vi "send_tmr2_rld.vi"(2 "error in (no error)":errorcluster, 3 "frekvencia":u16, 4 "VISA Refnum in":refnum<visa-resource-name>) -> (0 "error out":errorcluster, 1 "VISA Refnum out":refnum<visa-resource-name>)   [LabVIEW 2013]
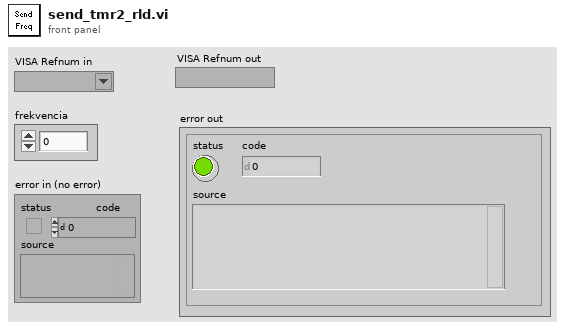
[diagram p1: front panel]
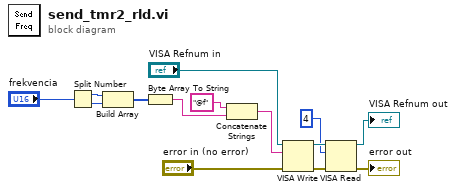
[diagram p0: block diagram]
diagram:
  n1 = Split Number(x="frekvencia") -> (hi(x)=w11:u8, lo(x)=w12:u8)
  n2 = Build Array(w11, w12) -> (w13:u8[])
  n3 = Byte Array To String(unsigned byte array=w13) -> (string=w14:string)
  n4 = Concatenate Strings("@f" ("write buffer"), w14) -> (w4:string)
  n5 = VISA Write(VISA resource name="VISA Refnum in", write buffer=w4, error in (no error)="error in (no error)") -> (VISA resource name out=w6:refnum<visa-resource-name>, error out=w7:errorcluster)  [unwired: 1 out]
  n6 = VISA Read(VISA resource name=w6, byte count=u32 4, error in (no error)=w7) -> (VISA resource name out=→"VISA Refnum out":refnum<visa-resource-name>, error out=→"error out":errorcluster)  [unwired: 2 out]
